vi "repPrepareKickoffEnemyPlay.vi"(8 "error in (no error)":errorcluster, 9 "Game in 2":refnum<class "Game.lvclass">, 10 "RobotPlacement":T1(array[cluster]), 11 "PrepareKickoffEnemyPlay in":refnum<class "PrepareKickoffEnemyPlay.lvclass">) -> (0 "error out":errorcluster, 2 "RobotPlacement 2":T1(array[cluster]), 3 "PrepareKickoffEnemyPlay out":refnum<class "PrepareKickoffEnemyPlay.lvclass">)   [LabVIEW 2020, in "PrepareKickoffEnemyPlay.lvclass"]
uses:
  PrepareKickoffEnemyPlay.lvclass
  Game_class/Game.lvclass
  Field_class/Field.lvclass
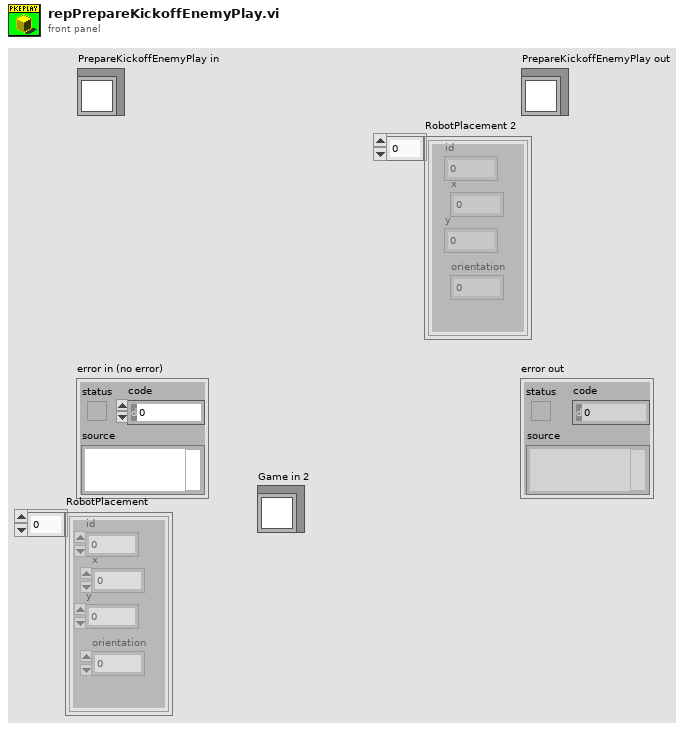
[diagram p1: front panel]
types:
  T1 = cluster{"id":i32, "x":dbl, "y":dbl, "orientation":dbl}[]
  T2 = cluster{"id":i32, "x":dbl, "y":dbl, "orientation":dbl}
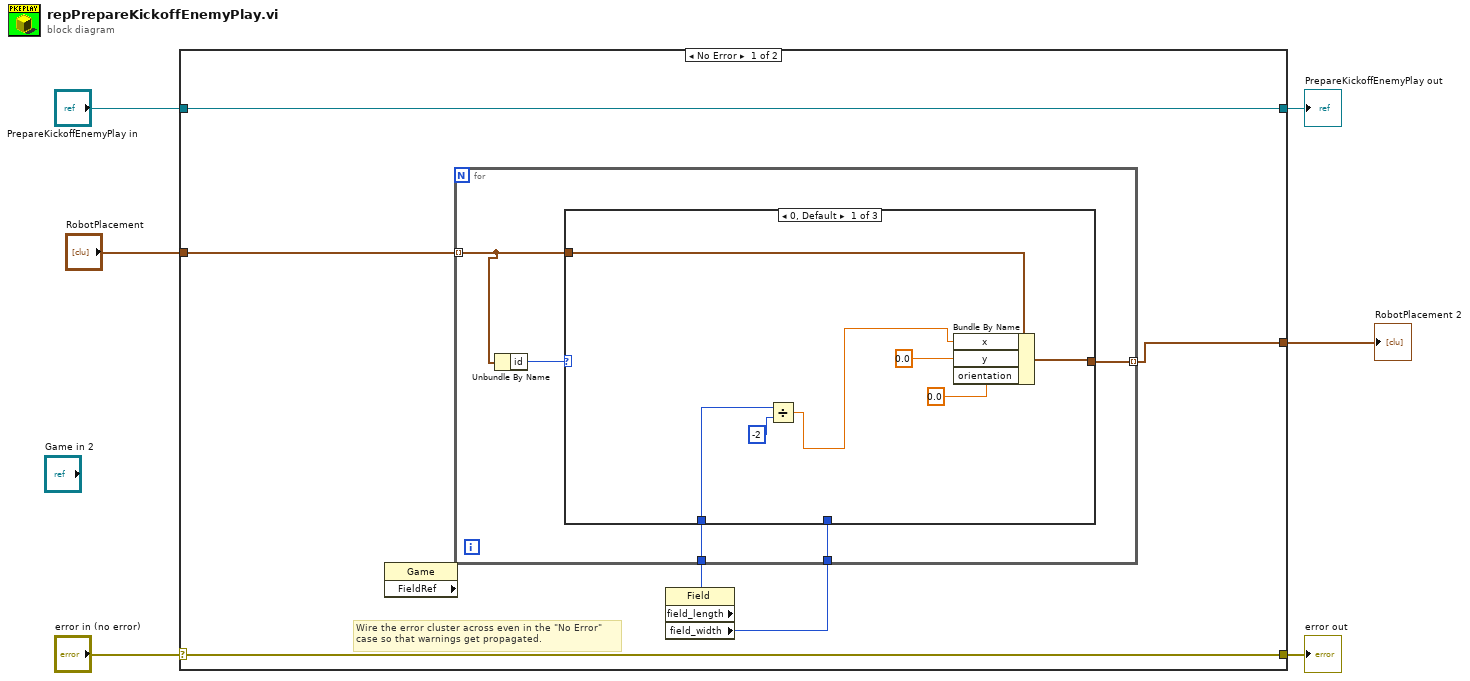
[diagram p0: block diagram]
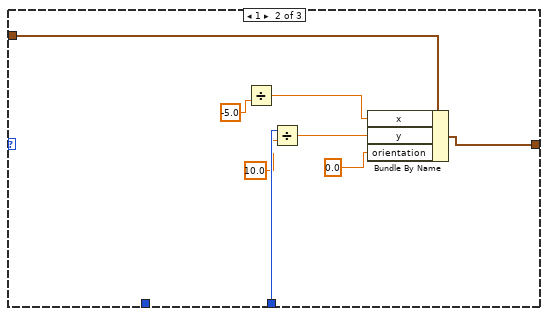
[diagram p2: hidden frame]
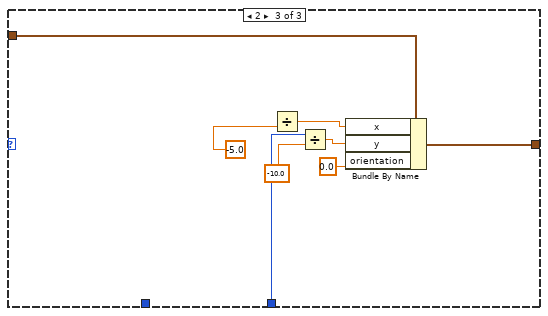
[diagram p3: hidden frame]
diagram:
  n1 = case shown="No Error" "error in (no error)" {
    selector: "error in (no error)" -> [w11 w42]
    tunnel: [w11 w42] -> w5
    tunnel: [w12 w41] -> w3
    tunnel: "PrepareKickoffEnemyPlay in" -> [w12 w41]
    tunnel: [w8 _] -> w2
    tunnel: "RobotPlacement" -> [w7 _]
    frame No Error {
      # "Wire the error cluster across even in the \"No Error\"\ncase so that warnings get propagated."
      n2 = property class="Game" props=["FieldRef"]() -> ()  [unwired: 2 in, 3 out]
      n3 = property class="Field"() -> ("field_length"=w10:i32, "field_width"=w9:i32)  [unwired: 2 in, 2 out]
      n4 = for {
        tunnel: [w17] -> w8 mode=indexing
        tunnel: w10 -> [w13]
        tunnel: w9 -> [w16]
        tunnel: w7 -> [w15] mode=indexing
        n5 = Unbundle By Name(w15) -> ("id"=w14:i32)
        n6 = case shown="0, Default" w14 {
          tunnel: [w24 w31 w40] -> w17
          tunnel: w16 -> [_ w30 w36]
          tunnel: w15 -> [w19 w25 w33]
          tunnel: w13 -> [w18 _ _]
          frame 0, Default {
            n7 = Divide(x=w18, y=-2) -> (x/y=w22:dbl)
            n8 = Bundle By Name(cluster=w19, "x"=w22, "y"=0.0, "orientation"=0.0) -> (w24:T2)
          }
          frame 1 {
            n9 = Divide(y=-5.0 ("x")) -> (x/y=w26:dbl)  [unwired: 1 in]
            n10 = Divide(x=w30, y=10.0 ("x")) -> (x/y=w27:dbl)
            n11 = Bundle By Name(cluster=w25, "x"=w26, "y"=w27, "orientation"=0.0 ("x")) -> (w31:T2)
          }
          frame 2 {
            n12 = Divide(y=-5.0 ("x")) -> (x/y=w34:dbl)  [unwired: 1 in]
            n13 = Divide(x=w36, y=-10.0 ("x")) -> (x/y=w35:dbl)
            n14 = Bundle By Name(cluster=w33, "x"=w34, "y"=w35, "orientation"=0.0) -> (w40:T2)
          }
        }
      }
    }
    frame Error {
    }
  }
  "error out" <- w5
  "PrepareKickoffEnemyPlay out" <- w3
  "RobotPlacement 2" <- w2
